vi "替换数组子集函数.vi"() -> ()   [LabVIEW 2014]
panel:
  out "输出数组 5":i32[][](array[numeric])
  out "输出数组 4":i32[][](array[numeric])
  out "输出数组 2":i32[][](array[numeric])
  out "输出数组":i32[][](array[numeric])
  out "输出数组 3":i32[][](array[numeric])
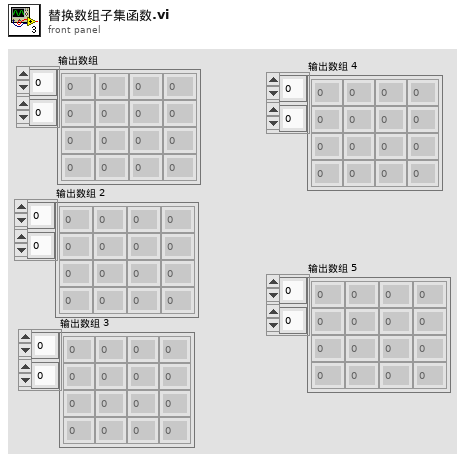
[diagram p1: front panel]
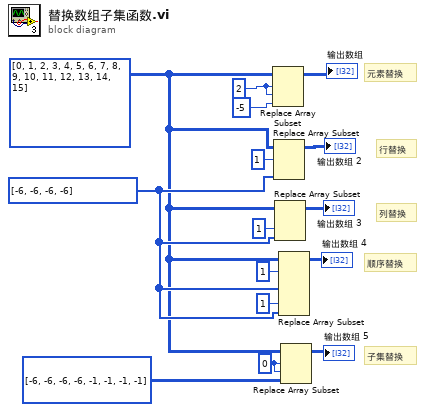
[diagram p0: block diagram]
diagram:
  w3 = 0 ("索引 (行)")
  w6 = i32[] [-6, -6, -6, -6]
  w4 = i32[][] [[0, 1, 2, 3], [4, 5, 6, 7], [8, 9, 10, 11], [12, 13, 14, 15]]
  w13 = 2 ("索引")
  # "子集替换"
  # "顺序替换"
  # "列替换"
  # "行替换"
  # "元素替换"
  n1 = Replace Array Subset(array=w4, new element=-5 ("新元素/子数组"), index (row)=w13, index (col)=w13) -> (→"输出数组":i32[][])
  n2 = Replace Array Subset(array=w4, new element=w6, index (row)=1 ("索引")) -> (→"输出数组 2":i32[][])  [unwired: 1 in]
  n3 = Replace Array Subset(array=w4, new element=w6, index (col)=1 ("禁用的索引 (列)")) -> (→"输出数组 3":i32[][])  [unwired: 1 in]
  n4 = Replace Array Subset(array=w4, new element #1=w6, index (row) #1=1 ("索引 (行)"), new element #2=w6, index (col) #2=1 ("禁用的索引 (列)")) -> (→"输出数组 4":i32[][])  [unwired: 2 in]
  n5 = Replace Array Subset(array=w4, new element=i32[][] [[-6, -6, -6, -6], [-1, -1, -1, -1]], index (row)=w3, index (col)=w3) -> (→"输出数组 5":i32[][])
